vi "BurstRead.vi"() -> ()   [LabVIEW 2016]
uses:
  <vilib>/Analysis/NI_AALPro.lvlib
panel:
  out "spec":waveform(dbl)[](graph)
  out "graph":waveform(dbl)[](graph)
  out "spec":waveform(dbl)[](graph)
  out "signal":dbl[][](graph)
  out "data":T1
  in  "File":path
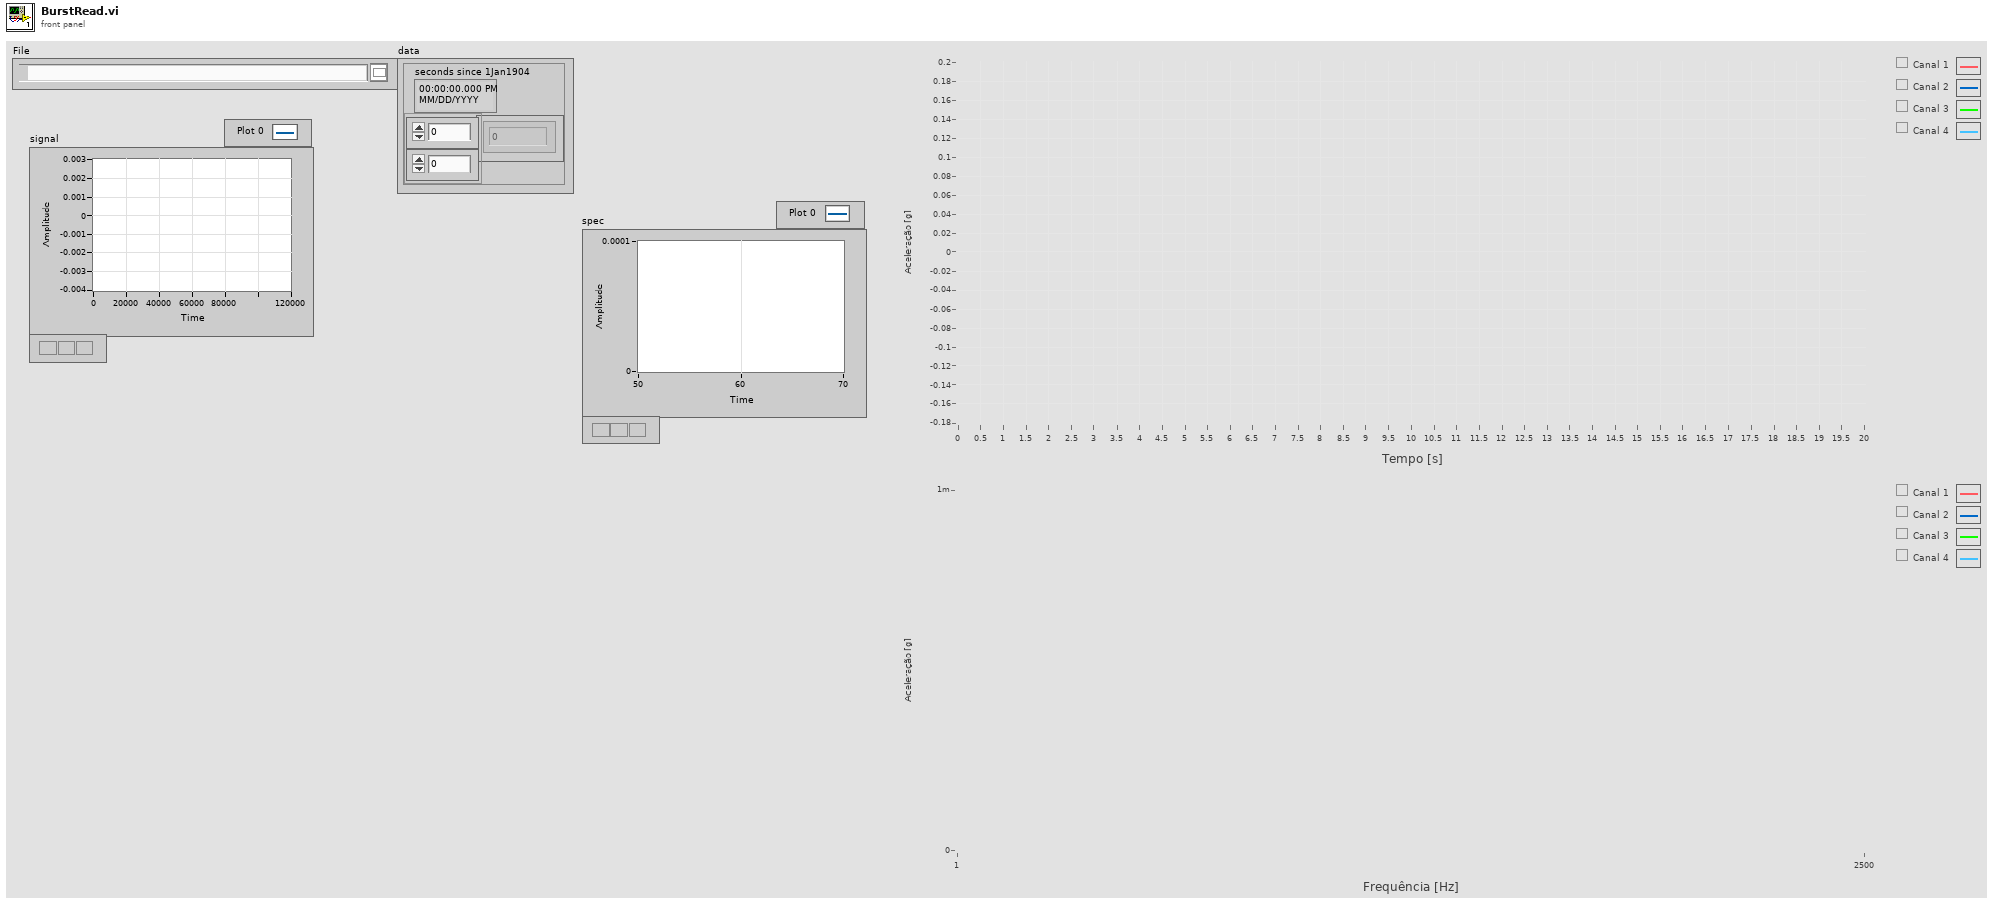
[diagram p1: front panel]
types:
  T1 = cluster{"seconds since 1Jan1904":timestamp, "Array":dbl[][]}
  T2 = cluster{"seconds since 1Jan1904":timestamp, dbl[][]}
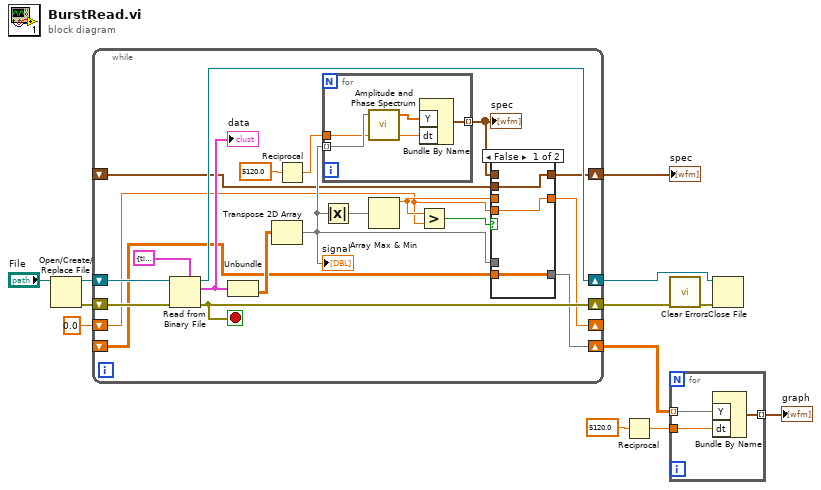
[diagram p0: block diagram]
diagram:
  n1 = Open/Create/Replace File(file path (use dialog)="File") -> (refnum out=w11:refnum<file>, error out=w10:errorcluster)  [unwired: 5 in, 1 out]
  n2 = while {
    shift-right: [w28] -> w8
    shift-left: w10 -> [w30]
    shift-right: [w29] -> w9
    shift-left: w11 -> [w32]
    shift-right: [w20] -> _
    shift-left: 0.0 -> [w13]
    shift-right: [w18] -> w1
    shift-left: _ -> [w14]
    shift-right: [w16] -> w5
    shift-left: _ -> [w15]
    stop <- w28 stop-if-true
    n3 = Read from Binary File(5:T2 {"seconds since 1Jan1904"=timestamp(0 s since 1904-01-01), []} ("output cluster"), 8:w30, 11:w32) -> (0:w28:errorcluster, 2:w27:T2, 3:w29:refnum<file>)  [unwired: 3 in, 1 out]
    "data" <- w27
    n4 = Unbundle(w27) -> (w26:dbl[][])  [unwired: 1 out]
    n5 = Transpose 2D Array(2D array=w26) -> (transposed array=w17:dbl[][])
    "signal" <- w17
    n6 = Reciprocal(x=5120.0) -> (1/x=w24:dbl)
    n7 = for {
      tunnel: w17 -> [w43] mode=indexing
      tunnel: w24 -> [w42]
      tunnel: [w39] -> w19 mode=indexing
      n8 = call <vilib>:"Amplitude and Phase Spectrum.vi"("dt"=w42, "Signal (V)"=w43) -> ("df"=w40:dbl, "Amp Spectrum Mag (Vrms)"=w41:dbl[])  [unwired: 1 in, 1 out]
      n9 = Bundle By Name("Y"=w41, "dt"=w40) -> (w39:waveform(dbl))  [unwired: 1 in]
    }
    "spec" <- w19
    n10 = Absolute Value(x=w17) -> (abs(x)=w23:dbl[][])
    n11 = Array Max & Min(array=w23) -> (max value=w21:dbl)  [unwired: 3 out]
    n12 = Greater?(x=w21, y=w13) -> (0:w22:bool)
    n13 = case shown="False" w22 {
      tunnel: w21 -> [_ w38]
      tunnel: [w33 w38] -> w20
      tunnel: w19 -> [_ w37]
      tunnel: [w34 w37] -> w18
      tunnel: w17 -> [_ w36]
      tunnel: [w35 w36] -> w16
      tunnel: w15 -> [w35 _]
      tunnel: w14 -> [w34 _]
      tunnel: w13 -> [w33 _]
      frame False {
      }
      frame True {
      }
    }
  }
  "spec" <- w1
  n14 = Reciprocal(x=5120.0) -> (1/x=w3:dbl)
  n15 = call <vilib>:"Clear Errors.vi"("error in (no error)"=w8) -> ("error out"=w7:errorcluster)  [unwired: 5 in, 1 out]
  n16 = for {
    tunnel: w5 -> [w45] mode=indexing
    tunnel: [w46] -> w2 mode=indexing
    tunnel: w3 -> [w44]
    n17 = Bundle By Name("Y"=w45, "dt"=w44) -> (w46:waveform(dbl))  [unwired: 1 in]
  }
  "graph" <- w2
  n18 = Close File(refnum=w9, error in=w7) -> ()  [unwired: 2 out]
